vi "Set Simple Numeric byPtr.vi"(4 "error in (no error)":errorcluster, 6 "Data":variant, 7 "Pointer":i32) -> (0 "error out":errorcluster, 3 "Duplicate Pointer":i32)   [LabVIEW 2011]
doc: "Use this VI to set any simple numeric value in memory using a pointer. The VI will return an error if anything other than a simple numeric value is wired to <B>Data</B>.\n\n*Warning - The Pointer VIs access memory directly. The VIs check for NULL pointers but may still cause access violations and crashes if used to access protected or otherwise inaccessible memory."
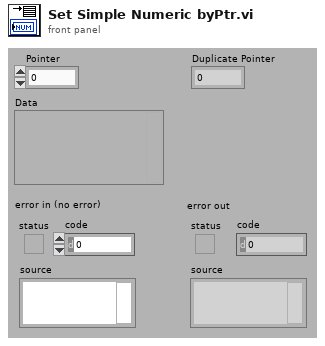
[diagram p1: front panel]
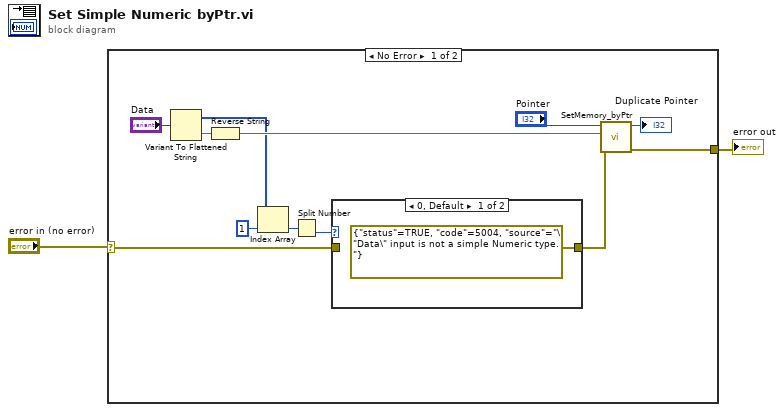
[diagram p0: block diagram]
diagram:
  n1 = case shown="No Error" "error in (no error)" {
    selector: "error in (no error)" -> [w3 w17]
    tunnel: [w4 w17] -> w2
    frame No Error {
      n2 = Variant To Flattened String(Variant="Data") -> (data string=w13:string, 1:w9:i16[])
      n3 = Reverse String(1:w13) -> (0:w12:string)
      n4 = Index Array(array=w9, index=1) -> (element=w7:i16)
      n5 = Split Number(x=w7) -> (lo(x)=w6:u8)  [unwired: 1 out]
      n6 = case shown="0, Default" w6 {
        tunnel: w3 -> [_ w16]
        tunnel: [errorcluster {"status"=TRUE, "code"=5004, "source"="\"Data\" input is not a simple Numeric type."} ("error in 2 (no error)") w16] -> w5
        frame 0, Default {
        }
        frame 1..11, 21..27 {
        }
      }
      n7 = call "SetMemory_byPtr.vi"("error in (no error)"=w5, "Input"=w12, "Pointer"="Pointer") -> ("error out"=w4:errorcluster, "Duplicate Pointer"=→"Duplicate Pointer":i32)  [unwired: 4 out]
    }
    frame Error {
    }
  }
  "error out" <- w2
